vi "Radar_4channel.vi"() -> ()   [LabVIEW 2014]
doc: "Personal Daq 54 example.\nTriggering is immediate and readings are returned 1 scan at a time as available.\nBe sure to use the Acquisition Stop control for proper shutdown."
uses:
  <vilib>/Utility/error.llb/DialogType.ctl
  <vilib>/DAQmx/read.llb/DAQmx Read (Analog 1D DBL NChan 1Samp).vi
  <vilib>/Analysis/2dsp.llb/Complex FFT.vi
  <vilib>/DAQmx/create/channels.llb/DAQmx Create Channel (AI-Voltage-Basic).vi
  <vilib>/DAQmx/configure/timing.llb/DAQmx Timing (Sample Clock).vi
  <vilib>/DAQmx/miscellaneous.llb/DAQmx Fill In Error Info.vi
  <vilib>/measure/madcrms.llb/Basic Averaged DC-RMS for 1 Chan.vi
  Instance          18 26Saved   noise_Nov07_2009_5 .vi
  <vilib>/measure/NI_MAPro.lvlib
  <vilib>/Analysis/NI_AALPro.lvlib
panel:
  out "Spectrum 2":waveform(dbl)(graph)
  out "I/Q Signal 2":dynamicdata(graph)
  out "I/Q Signal 1":dynamicdata(graph)
  in  "Save Data":bool
  in  "input terminal configuration":i32(ring)=10083 items=["default"=-1, "RSE"=10083, "NRSE"=10078, "Differential"=10106, "Pseudodifferential"=12529]
  in  "stop":bool
  in  "Maximum Value":dbl=5.0 format="%0.2f"
  in  "Minimum Value":dbl format="%0.2f"
  in  "Rate":dbl=20.0 caption="Sample Rate (Hz)" format="%0.2f"
  in  "Samples per Channel":i32=1
  out "Spectrum 1":waveform(dbl)(graph)
  in  "FFT":i32=256
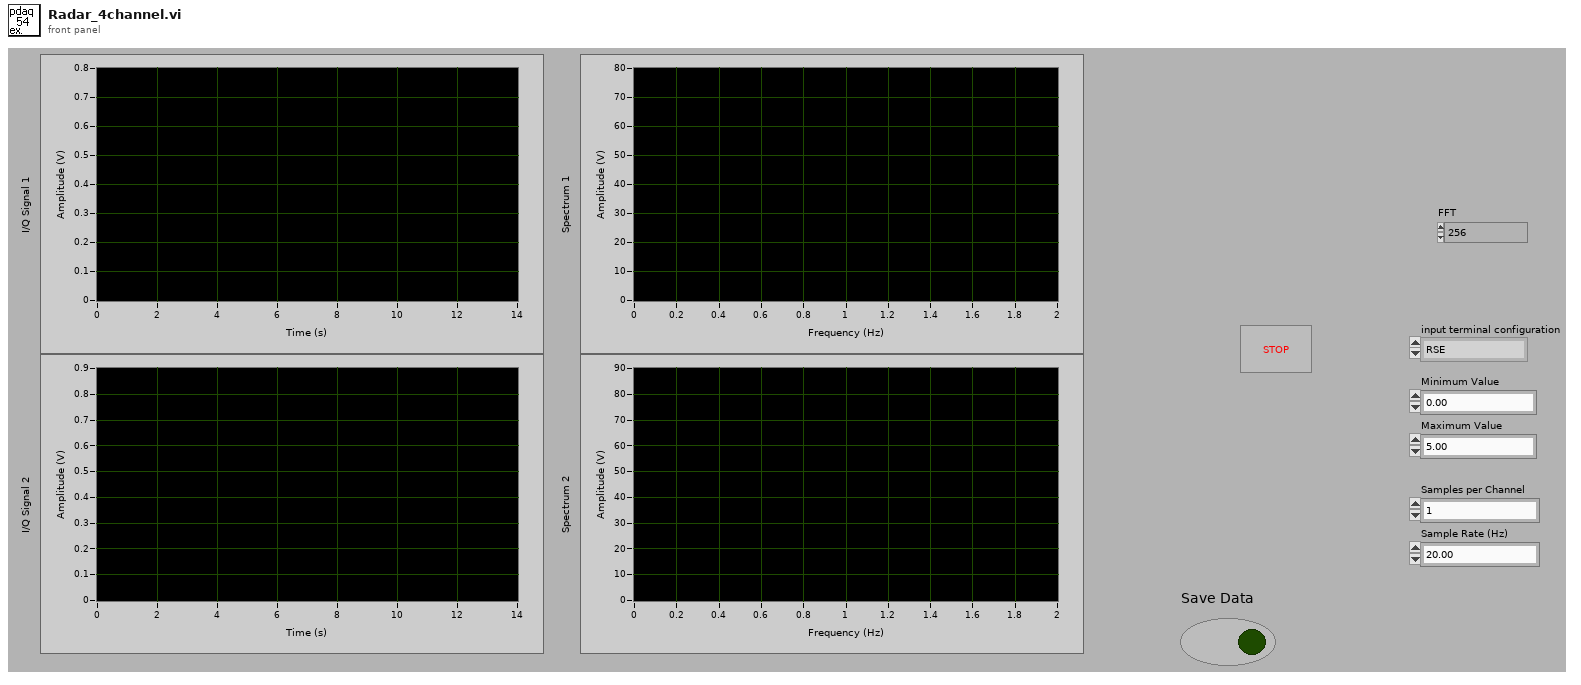
[diagram p1: front panel]
types:
  T1 = typedef "DialogType.ctl" = u16
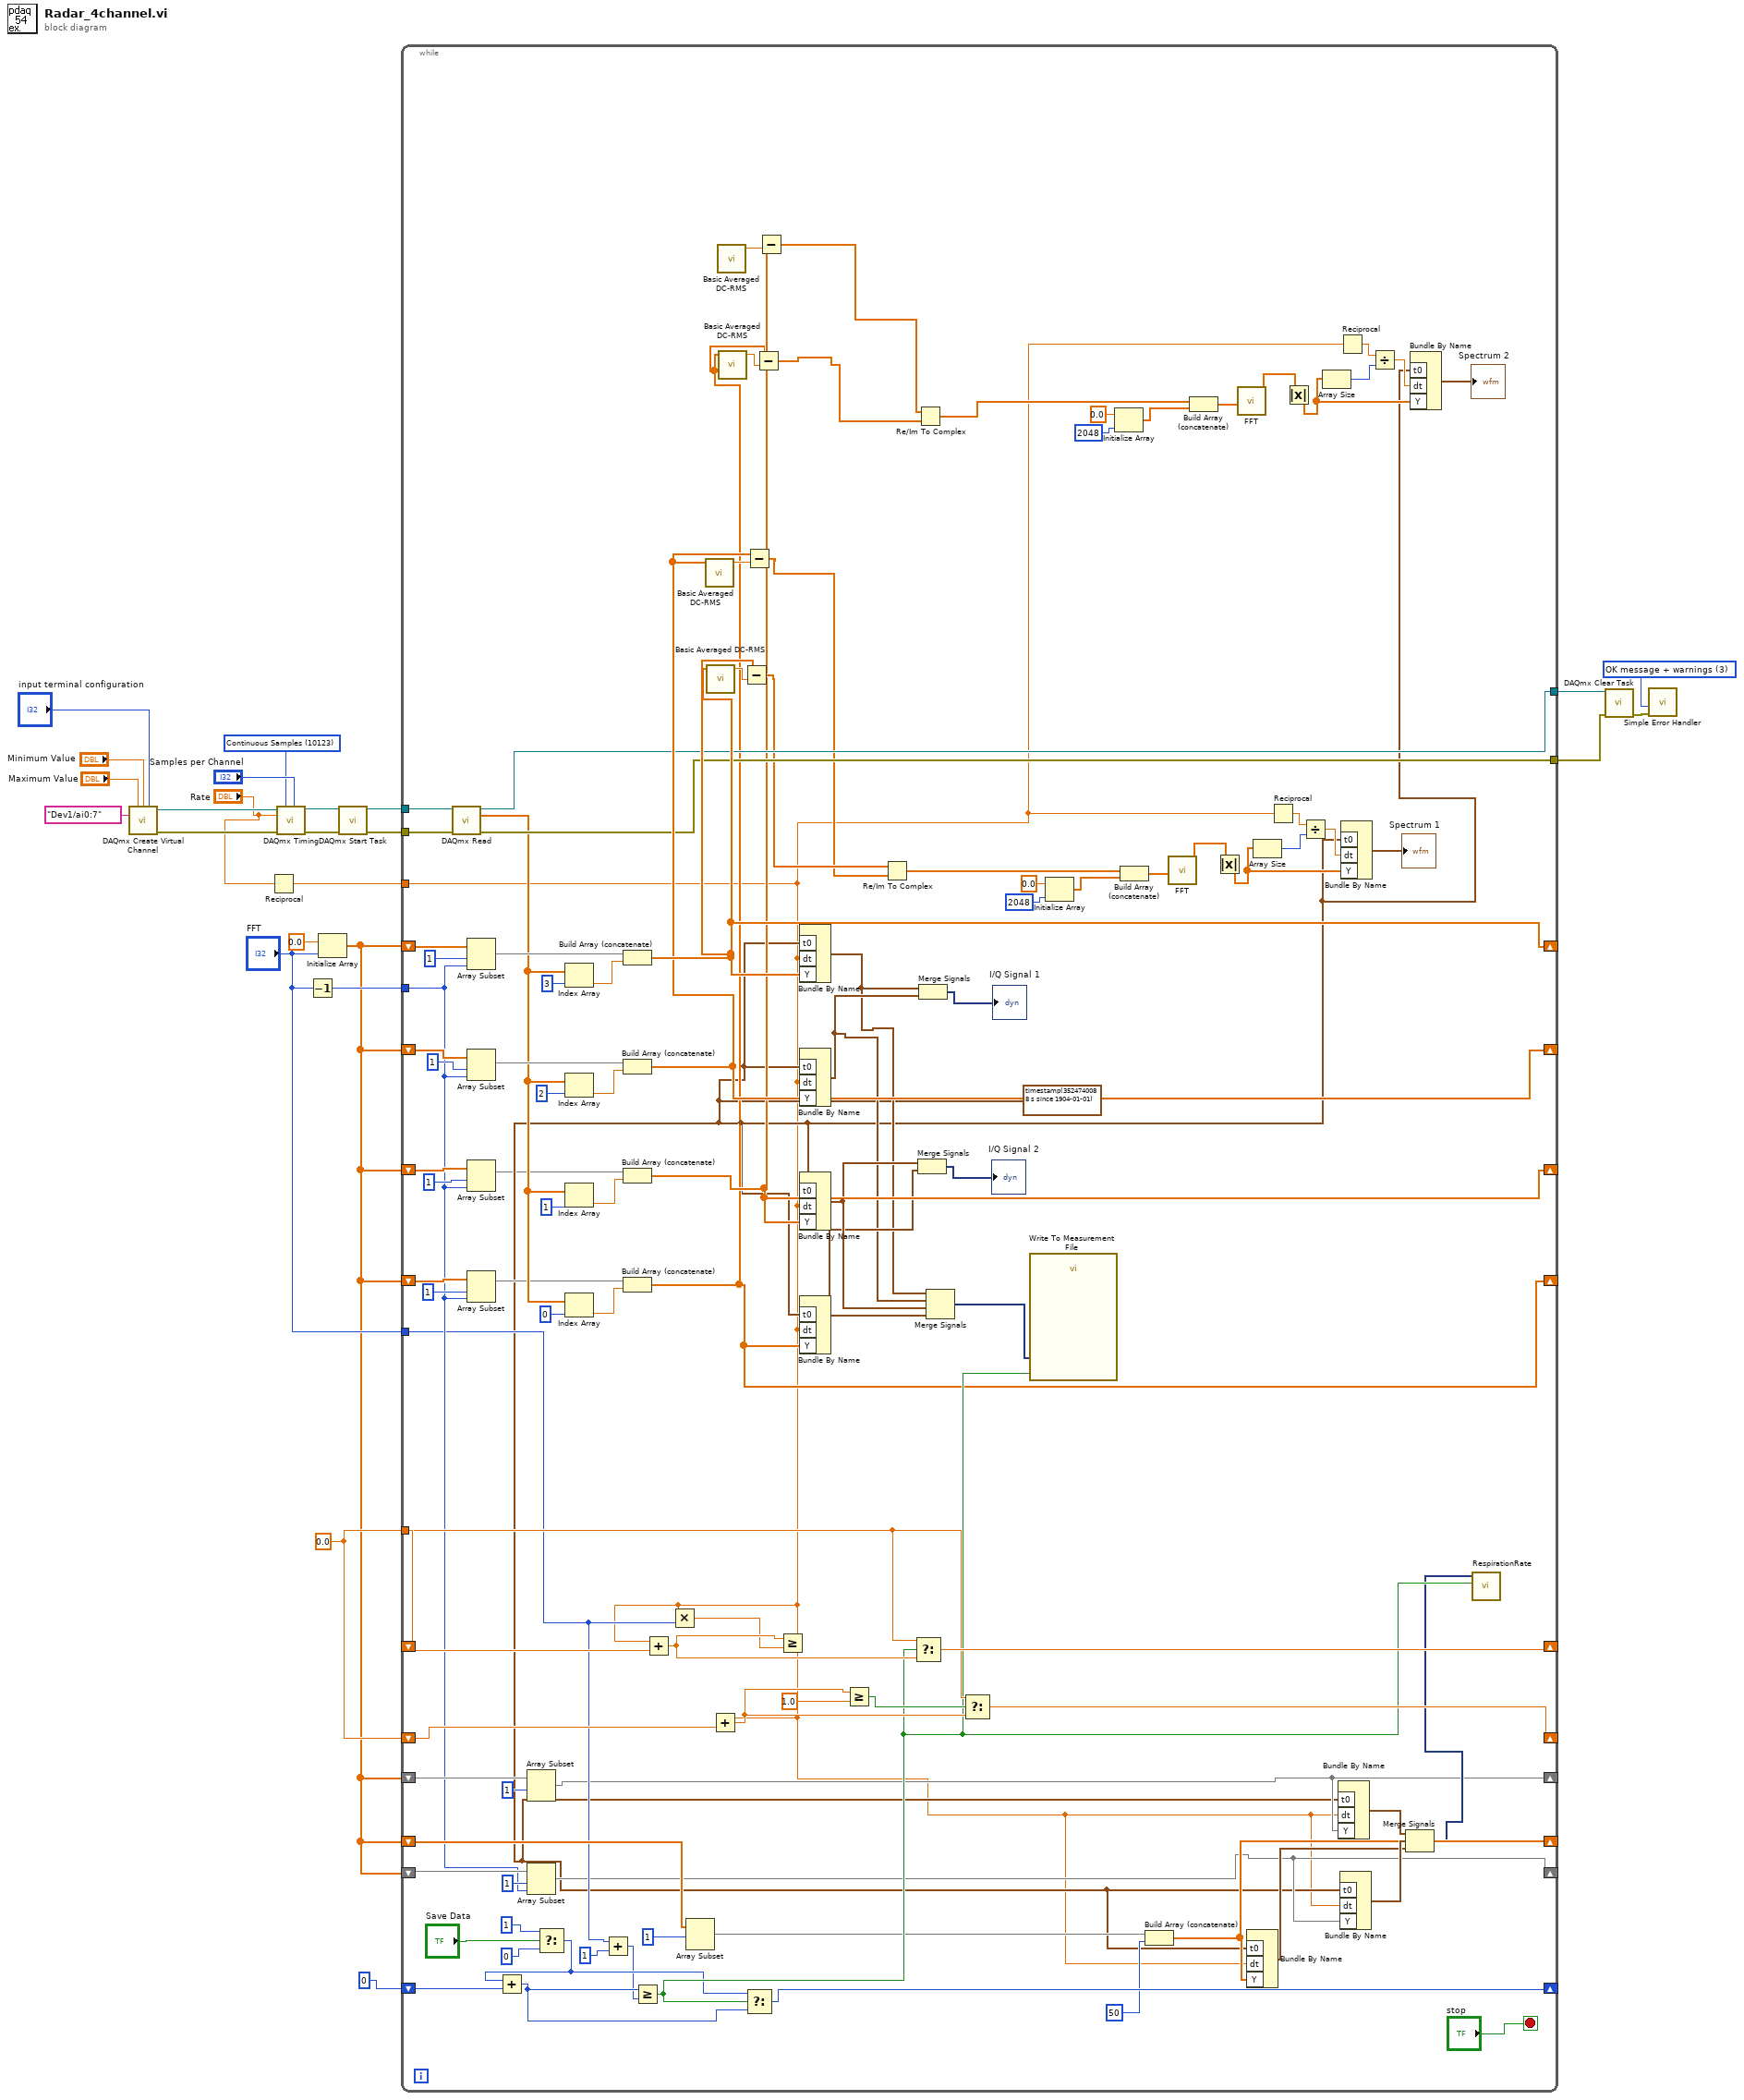
[diagram p0: block diagram]
diagram:
  w5 = 0.0 ("element")
  w11 = T1 3 items=["no dialog", "OK message", "continue or stop message", "OK message + warnings", "continue/stop + warnings"] ("type of dialog (OK msg:1)")
  w17 = 10123 items=["Finite Samples"=10178, "Continuous Samples"=10123] ("sample mode")
  n1 = call-poly <vilib>:"DAQmx Create Virtual Channel.vi"("maximum value"="Maximum Value", "minimum value"="Minimum Value", "input terminal configuration"="input terminal configuration", "physical channels"=tag "Dev1/ai0:7") -> ("task out"=w18:refnum<k21>, "error out"=w20:errorcluster)  [unwired: 5 in, 5 out]
  n2 = Reciprocal(x="Rate") -> (1/x=w2:dbl)
  n3 = call-poly <vilib>:"DAQmx Timing.vi"("task/channels in"=w18, "sample mode"=w17, "samples per channel"="Samples per Channel", "rate"="Rate", "error in"=w20) -> ("task out"=w16:refnum<k21>, "error out"=w15:errorcluster)  [unwired: 2 in, 7 out]
  n4 = Decrement(x="FFT") -> (x-1=w23:i32)
  n5 = Initialize Array(0.0 ("element"), "FFT") -> (w3:dbl[])
  n6 = call <vilib>:"DAQmx Start Task.vi"("task/channels in"=w16, "error in"=w15) -> ("task out"=w13:refnum<k21>, "error out"=w12:errorcluster)  [unwired: 12 out]
  n7 = while {
    shift-right: [w114] -> _
    shift-left: w3 -> [w129]
    tunnel: w23 -> [w66]
    shift-right: [w113] -> _
    shift-left: w3 -> [w126]
    tunnel: w13 -> [w112]
    tunnel: w12 -> [w111]
    tunnel: w2 -> [w25]
    tunnel: [w110] -> w10
    tunnel: [w109] -> w9
    shift-right: [w104] -> _
    shift-left: w5 -> [w102]
    tunnel: "FFT" -> [w61]
    tunnel: w5 -> [w96]
    shift-right: [w100] -> _
    shift-left: w5 -> [w97]
    shift-right: [w50] -> _
    shift-left: w3 -> [w94]
    shift-right: [w51] -> _
    shift-left: w3 -> [w92]
    shift-right: [w84] -> _
    shift-left: 0 -> [w86]
    shift-right: [w57] -> _
    shift-left: w3 -> [w77]
    shift-right: [w70] -> _
    shift-left: w3 -> [w74]
    shift-right: [w56] -> _
    shift-left: w3 -> [w68]
    stop <- "stop" stop-if-true
    w31 = timestamp(3524740088.296 s since 1904-01-01) ("t0")
    n8 = call-poly <vilib>:"DAQmx Read.vi"("task/channels in"=w112, "error in"=w111) -> ("task out"=w110:refnum<k21>, "data"=w64:dbl[], "error out"=w109:errorcluster)  [unwired: 11 out]
    n9 = Array Subset(array=w129, index=1, length=w66) -> (w127:dbl[])
    n10 = Array Subset(array=w126, index=1, length=w66) -> (w124:dbl[])
    n11 = Array Subset(array=w77, index=1, length=w66) -> (w26:dbl[])
    n12 = Array Subset(array=w68, index=1, length=w66) -> (w63:dbl[])
    n13 = Array Subset(array=w92, index=1) -> (w51:dbl[])  [unwired: 1 in]
    n14 = Array Subset(array=w94, index=1, length=w66) -> (w50:dbl[])
    n15 = Select(t=1, s="Save Data", f=0) -> (s? t:f=w80:i32)
    n16 = Add(x=w80, y=w86) -> (x+y=w85:i32)
    n17 = Index Array(array=w64, index=3 ("index (row)")) -> (element=w30:dbl)
    n18 = Index Array(array=w64, index=2 ("index (row)")) -> (element=w29:dbl)
    n19 = Index Array(array=w64, index=1 ("index (row)")) -> (element=w28:dbl)
    n20 = Index Array(array=w64, index=0 ("index (row)")) -> (element=w27:dbl)
    n21 = Add(x=w61, y=1 ("index")) -> (x+y=w60:i32)
    n22 = Build Array (concatenate)(w127, w30) -> (w114:dbl[])
    n23 = Build Array (concatenate)(w124, w29) -> (w113:dbl[])
    n24 = Build Array (concatenate)(w26, w28) -> (w57:dbl[])
    n25 = Build Array (concatenate)(w63, w27) -> (w56:dbl[])
    n26 = Greater Or Equal?(x=w85, y=w60) -> (x >= y?=w83:bool)
    n27 = Add(x=w25, y=w102) -> (x+y=w105:dbl)
    n28 = Multiply(x=w25, y=w61) -> (x*y=w103:dbl)
    n29 = Array Subset(array=w74, index=1) -> (w72:dbl[])  [unwired: 1 in]
    n30 = call-poly <vilib>:"Basic Averaged DC-RMS.vi"("signal in"=w113) -> ("DC value"=w120:dbl)  [unwired: 4 in, 6 out]
    n31 = call-poly <vilib>:"Basic Averaged DC-RMS.vi"("signal in"=w114) -> ("DC value"=w119:dbl)  [unwired: 4 in, 6 out]
    n32 = Add(x=w25, y=w97) -> (x+y=w101:dbl)
    n33 = call-poly <vilib>:"Basic Averaged DC-RMS.vi"("signal in"=w57) -> ("DC value"=w58:dbl)  [unwired: 4 in, 6 out]
    n34 = call-poly <vilib>:"Basic Averaged DC-RMS.vi"("signal in"=w56) -> ("DC value"=w59:dbl)  [unwired: 4 in, 6 out]
    n35 = Subtract(x=w114, y=w119) -> (x-y=w107:dbl[])
    n36 = Subtract(x=w113, y=w120) -> (x-y=w106:dbl[])
    n37 = Select(t=w80, s=w83, f=w85) -> (s? t:f=w84:i32)
    n38 = Subtract(x=w56, y=w59) -> (x-y=w55:dbl[])
    n39 = Subtract(x=w57, y=w58) -> (x-y=w54:dbl[])
    n40 = Greater Or Equal?(x=w105, y=w103) -> ()  [unwired: 1 out]
    n41 = Bundle By Name("t0"=w31, "dt"=w25, "Y"=w114) -> (w44:waveform(dbl))  [unwired: 1 out]
    n42 = Bundle By Name("t0"=w31, "dt"=w25, "Y"=w113) -> (w45:waveform(dbl))  [unwired: 1 out]
    n43 = Bundle By Name("t0"=w31, "dt"=w25, "Y"=w57) -> (w47:waveform(dbl))  [unwired: 1 out]
    n44 = Bundle By Name("t0"=w31, "dt"=w25, "Y"=w56) -> (w46:waveform(dbl))  [unwired: 1 out]
    n45 = Greater Or Equal?(x=w101, y=1.0) -> (x >= y?=w98:bool)
    n46 = Re/Im To Complex(1:w106, 2:w107) -> (0:w121:cdb[])
    n47 = Select(t=w96, s=w83, f=w105) -> (s? t:f=w104:dbl)
    n48 = Re/Im To Complex(1:w55, 2:w54) -> (0:w32:cdb[])
    n49 = Merge Signals(w47, w46) -> (→"I/Q Signal 2":dynamicdata)
    n50 = Merge Signals(w44, w45) -> (→"I/Q Signal 1":dynamicdata)
    n51 = Merge Signals(w44, w45, w47, w46) -> (w43:dynamicdata)
    n52 = Select(t=w96, s=w98, f=w101) -> (s? t:f=w100:dbl)
    n53 = call "Write To Measurement File"("Signals"=w43, "Enable"=w83) -> ()  [unwired: 15 in, 3 out]
    n54 = Initialize Array(0.0 ("element"), 2048 ("dimension size")) -> (w53:dbl[])
    n55 = Initialize Array(0.0 ("element"), 2048 ("dimension size")) -> (w42:dbl[])
    n56 = Build Array (concatenate)(w121, w53) -> (w115:cdb[])
    n57 = Build Array (concatenate)(w72, 50 ("index")) -> (w70:dbl[])
    n58 = call-poly <vilib>:"FFT.vi"("X"=w115) -> ("FFT {X}"=w118:cdb[])  [unwired: 2 in, 8 out]
    n59 = Build Array (concatenate)(w32, w42) -> (w37:cdb[])
    n60 = Absolute Value(x=w118) -> (abs(x)=w78:dbl[])
    n61 = call-poly <vilib>:"FFT.vi"("X"=w37) -> ("FFT {X}"=w34:cdb[])  [unwired: 2 in, 8 out]
    n62 = Bundle By Name("t0"=w31, "dt"=w25, "Y"=w70) -> (w71:waveform(dbl))  [unwired: 1 out]
    n63 = Array Size(array=w78) -> (size(s)=w116:i32)
    n64 = Reciprocal(x=w25) -> (1/x=w88:dbl)
    n65 = Absolute Value(x=w34) -> (abs(x)=w41:dbl[])
    n66 = Divide(x=w88, y=w116) -> (x/y=w87:dbl)
    n67 = Array Size(array=w41) -> (size(s)=w36:i32)
    n68 = Reciprocal(x=w25) -> (1/x=w39:dbl)
    n69 = Bundle By Name("t0"=w31, "dt"=w25, "Y"=w51) -> (w91:waveform(dbl))  [unwired: 1 out]
    n70 = Bundle By Name("t0"=w31, "dt"=w25, "Y"=w50) -> (w90:waveform(dbl))  [unwired: 1 out]
    n71 = Bundle By Name("t0"=w31, "dt"=w87, "Y"=w78) -> (→"Spectrum 1":waveform(dbl))  [unwired: 1 out]
    n72 = Divide(x=w39, y=w36) -> (x/y=w40:dbl)
    n73 = Merge Signals(w91, w90, w71) -> (w52:dynamicdata)
    n74 = Bundle By Name("t0"=w31, "dt"=w40, "Y"=w41) -> (→"Spectrum 2":waveform(dbl))  [unwired: 1 out]
    n75 = call "RespirationRate"("Enable"=w83, "Signals"=w52) -> ()  [unwired: 3 in, 7 out]
  }
  n76 = call <vilib>:"DAQmx Clear Task.vi"("task in"=w10, "error in"=w9) -> ("error out"=w8:errorcluster)  [unwired: 13 out]
  n77 = call <vilib>:"Simple Error Handler.vi"("type of dialog (OK msg:1)"=w11, "error in (no error)"=w8) -> ()  [unwired: 8 out]
